vi "Control - Intake Air Measured.vi"(0 "MEP Desired [bar] (MAF w/ EGR Only)":sgl, 5 "Fuel [mg/cyc] (Fdbk)":sgl, 7 "Fuel Trim Integral Effort [mg/cyc] (VE Learn) (Fdbk) (optional)":sgl, 9 "Pre-Calculated EGR Mass Flow [kg/hr] (MAP Only)":sgl, 11 "Control Inputs":T1={"Engine Speed [RPM]"=0.0, "Engine Status"=enum."STALLED", "Load Control \nMode"=enum."High-Idle Governor", "dt(s)"=0.0, "Number of Cylinders"=0, "Engine Displacement [cc]"=0.0, "StoichAFR"=0.0, "Q.LHV Fuel [kJ/kg]"=0.0, "BattV PSU [V]"=0.0, "12V PSU [V]"=0.0, "5V PSU [V]"=0.0, "Pedal Position [%]"=0.0, "Oil Pressure [kPa]"=0.0, "Oil Temp [C]"=0.0, "Oil Level [%]"=0.0, "Engine Coolant Temp (ECT) [C]"=0.0, "Engine Coolant Pressure [kPa]"=0.0, "Rail Pressure [bar]"=0.0, "Fuel Pressure [kPa]"=0.0, "Fuel Temp [C]"=0.0, "Vacuum Pressure [kPa]"=0.0, "Throttle Position [%]"=0.0, "Cam1 Advance [CAD]"=0.0, "Cam2 Advance [CAD]"=0.0, "Cam3 Advance [CAD]"=0.0, "Cam4 Advance [CAD]"=0.0, "CA50 Control Output [CAD]"=[], "CA50 Control Output Valid"=[], "Intake Air Temp (IAT) [C]"=0.0, "Barometric Air Pressure [kPa]"=0.0, "Intake Air Rel. Humidity [%]"=0.0, "Mass Air Flow (MAF) [kg/hr]"=0.0, "Turbo Inlet Air Pressure [kPa]"=0.0, "Turbo Inlet Air Temp [C]"=0.0, "Turbo Outlet Air Pressure [kPa]"=0.0, "Turbo Outlet Air Temp [C]"=0.0, "CAC Outlet Pressure [kPa]"=0.0, "CAC Outlet Temp [C]"=0.0, "Intake Manifold Pressure (MAP) [kPa]"=0.0, "Intake Manifold Temp (MAT) [C]"=0.0, "Exhaust Manifold Pressure [kPa]"=0.0, "Exhaust Manifold Temp [C]"=0.0, "HighP EGR Cooler Outlet Pressure [kPa]"=0.0, "HighP EGR Cooler Outlet Temp [C]"=0.0, "HighP EGR Differential Pressure [kPa]"=0.0, "HighP EGR Valve Position [%]"=0.0, "Turbo Outlet Exhaust Pressure [kPa]"=0.0, "Turbo Outlet Exhaust Temp [C]"=0.0, "VGT Position 1 [%]"=0.0, "VGT Position 2 [%]"=0.0, "Turbo Speed 1 [RPM]"=0.0, "Turbo Speed 2 [RPM]"=0.0, "LowP EGR Differential Pressure [kPa]"=0.0, "LowP EGR Valve Position [%]"=0.0, "UEGO1Lambda"=0.0, "UEGO1_Hot"=FALSE, "UEGO2Lambda"=0.0, "UEGO2_Hot"=FALSE, "Knock Intensity"=[], "Knock"=[]} {"Knock Intensity" format="%.2f"; "CA50 Control Output [CAD]" format="%.2f"; "Exhaust Manifold Temp [C]" format="%#_6f"; "UEGO2Lambda" format="%.2f"; "Intake Manifold Temp (MAT) [C]" format="%#_6f"; "UEGO1Lambda" format="%.2f"}) -> (4 "Volumetric Efficiency [%]":sgl, 6 "Available Air Mass [mg/cyc]":sgl, 8 "Fresh Air Mass [mg/cyc]":sgl, 10 "Intake Charge Mass [mg/cyc]":sgl, 15 "EGR Mass [mg/cyc]":sgl)   [LabVIEW 2015, in "ECS-RT.lvlib"]
uses:
  ECS-RT.lvlib
  Typedefs/Control Inputs/Control Inputs.ctl
  Typedefs/EPT/Engine Status.ctl
  Typedefs/MISC/Load Control Mode.ctl
  Typedefs/MISC/Intake Charge Mode.ctl
  ECS-Shared.lvlib
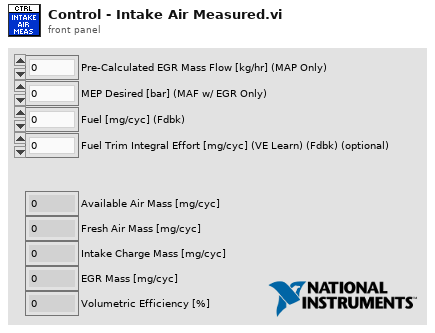
[diagram p1: front panel]
types:
  T1 = typedef "ECS-Shared.lvlib/Control Inputs.ctl" = cluster{"Engine Speed [RPM]":sgl, "Engine Status":T2, "Load Control \nMode":T3, "dt(s)":sgl, "Number of Cylinders":u8, "Engine Displacement [cc]":sgl, "StoichAFR":sgl, "Q.LHV Fuel [kJ/kg]":sgl, "BattV PSU [V]":sgl, "12V PSU [V]":sgl, "5V PSU [V]":sgl, "Pedal Position [%]":sgl, "Oil Pressure [kPa]":sgl, "Oil Temp [C]":sgl, "Oil Level [%]":sgl, "Engine Coolant Temp (ECT) [C]":sgl, "Engine Coolant Pressure [kPa]":sgl, "Rail Pressure [bar]":sgl, "Fuel Pressure [kPa]":sgl, "Fuel Temp [C]":sgl, "Vacuum Pressure [kPa]":sgl, "Throttle Position [%]":sgl, "Cam1 Advance [CAD]":sgl, "Cam2 Advance [CAD]":sgl, "Cam3 Advance [CAD]":sgl, "Cam4 Advance [CAD]":sgl, "CA50 Control Output [CAD]":sgl[], "CA50 Control Output Valid":bool[], "Intake Air Temp (IAT) [C]":sgl, "Barometric Air Pressure [kPa]":sgl, "Intake Air Rel. Humidity [%]":sgl, "Mass Air Flow (MAF) [kg/hr]":sgl, "Turbo Inlet Air Pressure [kPa]":sgl, "Turbo Inlet Air Temp [C]":sgl, "Turbo Outlet Air Pressure [kPa]":sgl, "Turbo Outlet Air Temp [C]":sgl, "CAC Outlet Pressure [kPa]":sgl, "CAC Outlet Temp [C]":sgl, "Intake Manifold Pressure (MAP) [kPa]":sgl, "Intake Manifold Temp (MAT) [C]":sgl, "Exhaust Manifold Pressure [kPa]":sgl, "Exhaust Manifold Temp [C]":sgl, "HighP EGR Cooler Outlet Pressure [kPa]":sgl, "HighP EGR Cooler Outlet Temp [C]":sgl, "HighP EGR Differential Pressure [kPa]":sgl, "HighP EGR Valve Position [%]":sgl, "Turbo Outlet Exhaust Pressure [kPa]":sgl, "Turbo Outlet Exhaust Temp [C]":sgl, "VGT Position 1 [%]":sgl, "VGT Position 2 [%]":sgl, "Turbo Speed 1 [RPM]":sgl, "Turbo Speed 2 [RPM]":sgl, "LowP EGR Differential Pressure [kPa]":sgl, "LowP EGR Valve Position [%]":sgl, "UEGO1Lambda":sgl, "UEGO1_Hot":bool, "UEGO2Lambda":sgl, "UEGO2_Hot":bool, "Knock Intensity":sgl[], "Knock":bool[]}
  T2 = typedef "ECS-Shared.lvlib/Engine Status.ctl" = enum16{"OFF", "STALLED", "CRANKING", "RUNNING", "ACCEL", "DECEL", "SAFE"}
  T3 = typedef "ECS-Shared.lvlib/Load Control Mode.ctl" = enum16{"No Governor", "Low-Idle Governor", "High-Idle Governor"}
  T4 = typedef "ECS-Shared.lvlib/Intake Charge Mode.ctl" = enum32{"MAF Only (No EGR)", "MAF Only (EGR)", "MAP Only (No EGR)", "MAP Only (EGR)", "MAF + MAP (EGR)"}
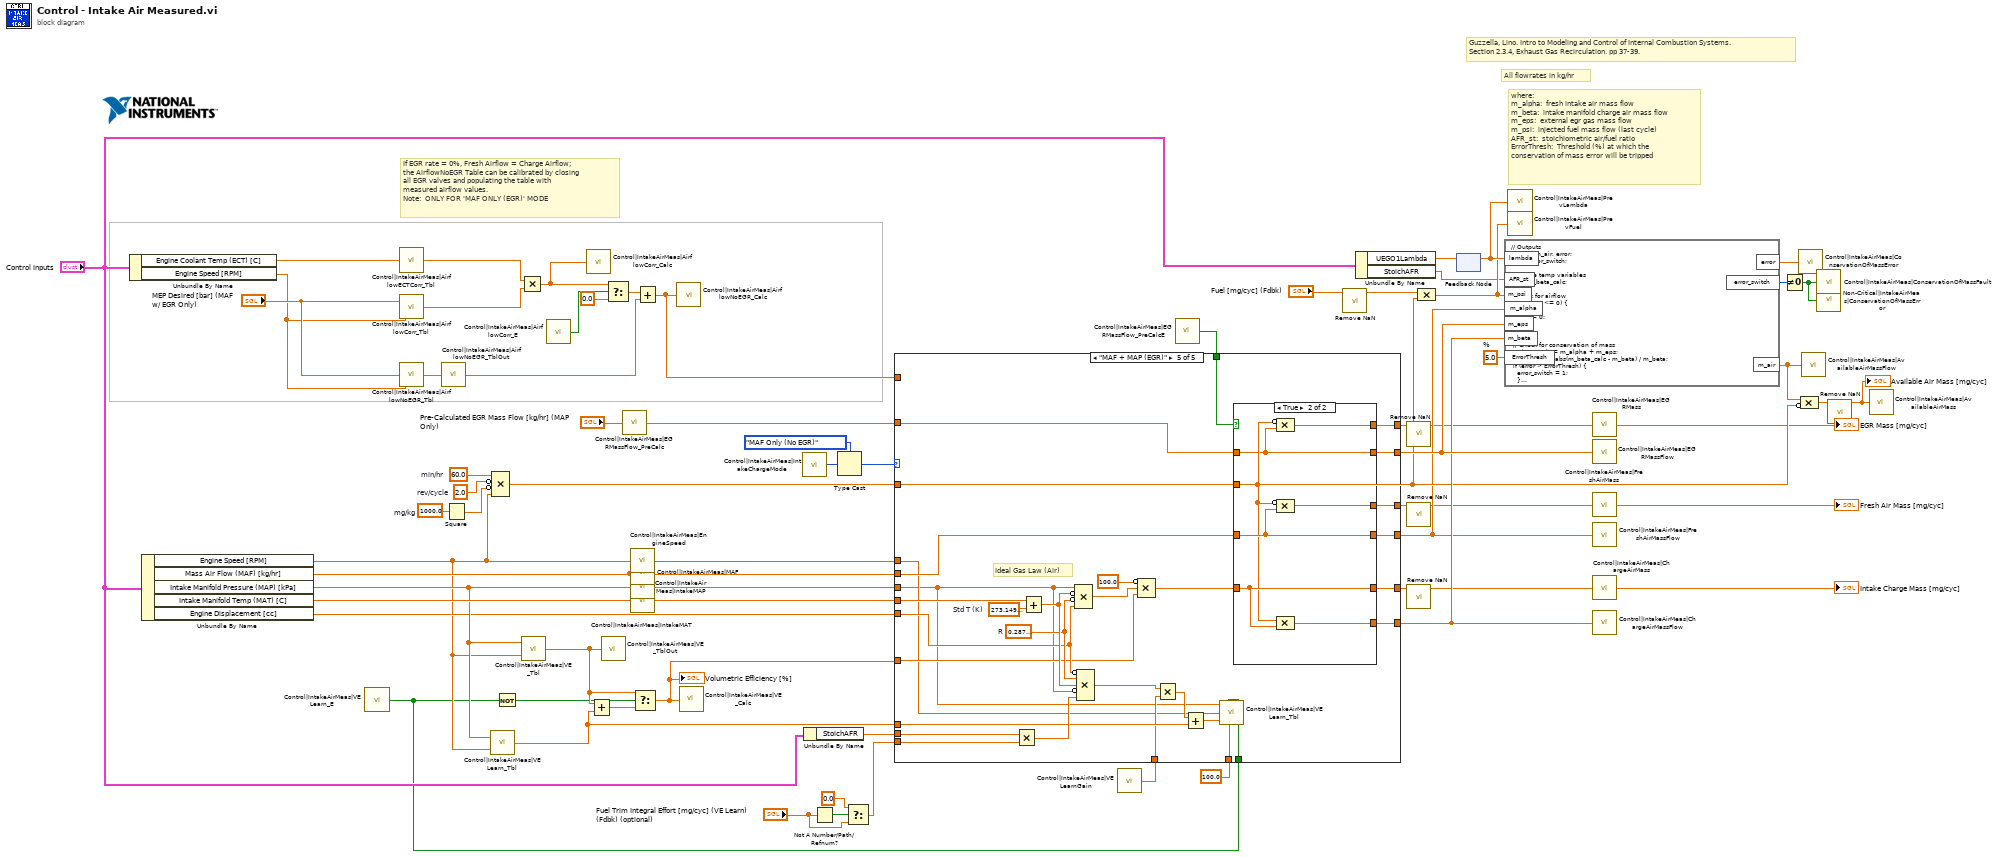
[diagram p0: block diagram]
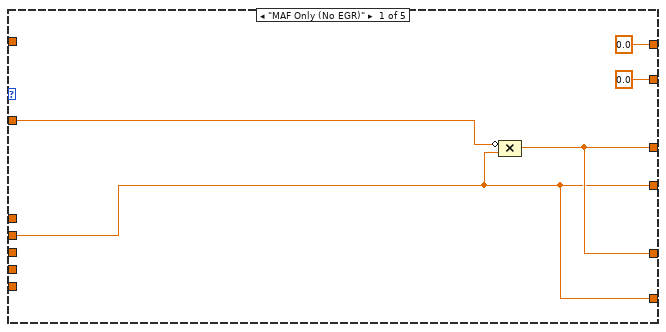
[diagram p2: hidden frame]
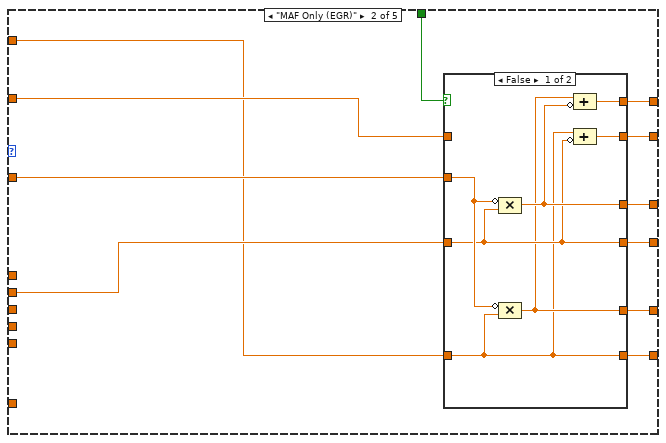
[diagram p3: hidden frame]
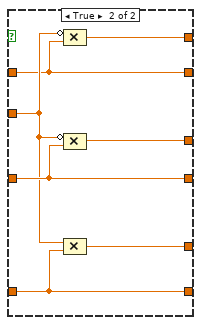
[diagram p4: hidden frame]
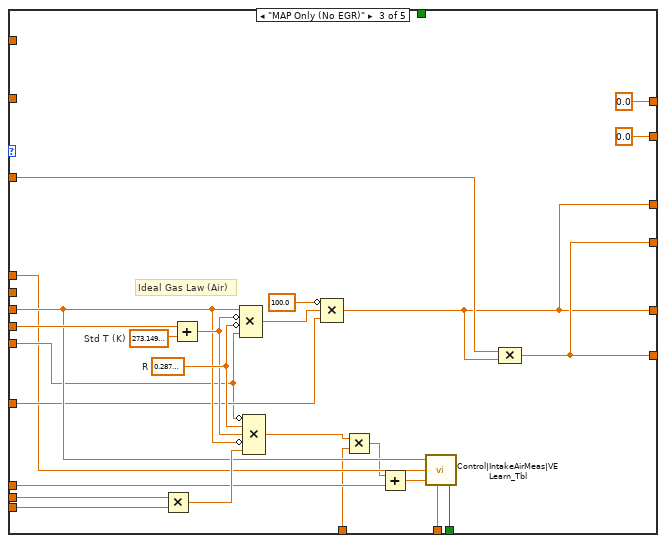
[diagram p5: hidden frame]
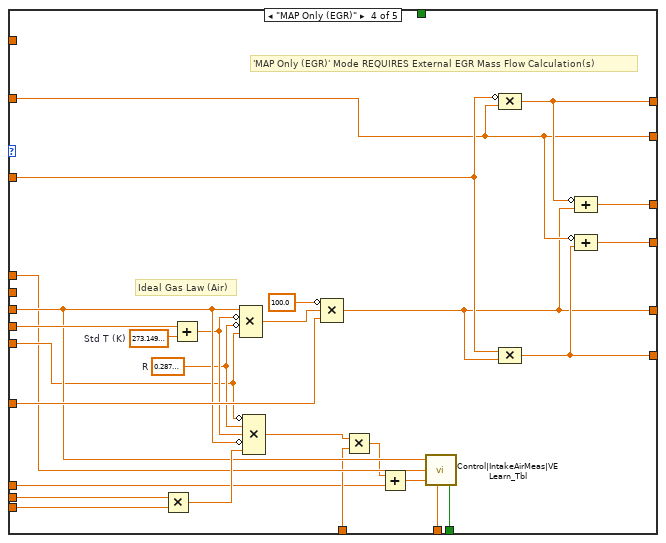
[diagram p6: hidden frame]
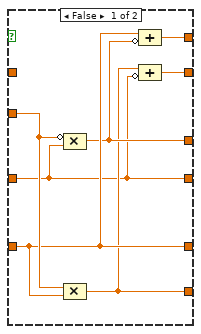
[diagram p7: hidden frame]
diagram:
  w40 = 5.0  # %
  w47 = sgl 60.0  # min/hr
  w48 = sgl 2.0  # rev/cycle
  w46 = sgl 1000.0  # mg/kg
  # "where:\nm_alpha:  fresh intake air mass flow\nm_beta:  intake manifold charge air mass flow\nm_eps:  external egr gas mass flow\nm_psi:  injected fuel mass flow (last cycle)\nAFR_st:  stoichiometric air/fuel ratio\nErrorThresh:  Threshold (%) at which the\nconservation of mass error will be tripped"
  # "All flowrates in kg/hr"
  # "Guzzella, Lino. Intro to Modeling and Control of Internal Combustion Systems.  \nSection 2.3.4, Exhaust Gas Recirculation. pp 37-39."
  # "If EGR rate = 0%, Fresh Airflow = Charge Airflow;\nthe AirflowNoEGR Table can be calibrated by closing\nall EGR valves and populating the table with\nmeasured airflow values.\nNote:  ONLY FOR 'MAF ONLY (EGR)' MODE"
  n1 = Unbundle By Name("Control Inputs") -> ("Engine Coolant Temp (ECT) [C]"=w52:sgl, "Engine Speed [RPM]"=w45:sgl)
  n2 = Unbundle By Name("Control Inputs") -> ("Engine Speed [RPM]"=w27:sgl, "Mass Air Flow (MAF) [kg/hr]"=w36:sgl, "Intake Manifold Pressure (MAP) [kPa]"=w29:sgl, "Intake Manifold Temp (MAT) [C]"=w35:sgl, "Engine Displacement [cc]"=w28:sgl)
  n3 = call "Control|IntakeAirMeas|VELearn_E"() -> ("Value"=w4:bool)
  n4 = call "Control|IntakeAirMeas|AirflowECTCorr_Tbl"("X Index"=w52) -> ("Y"=w57:sgl)
  n5 = call "Control|IntakeAirMeas|AirflowCorr_Tbl"("Y Index"=w45, "X Index"="MEP Desired [bar] (MAF w/ EGR Only)") -> ("Z"=w56:sgl)
  n6 = call "Control|IntakeAirMeas|AirflowNoEGR_Tbl"("Y Index"=w45, "X Index"="MEP Desired [bar] (MAF w/ EGR Only)") -> ("Z"=w59:sgl)
  n7 = call "Control|IntakeAirMeas|AirflowNoEGR_TblOut"("Value"=w59) -> ()
  n8 = Square(x=w46) -> (x^2=w49:sgl)
  n9 = call "Control|IntakeAirMeas|VELearn_Tbl"("Y Index"=w27, "X Index"=w29) -> ("Z"=w5:sgl)
  n10 = Compound Arithmetic op=MULTIPLY(w47, invert w48, invert w49, w27) -> (w26:sgl)
  n11 = Not(x=w4) -> (.not. x?=w3:bool)
  n12 = Multiply(x=w57, y=w56) -> (x*y=w58:sgl)
  n13 = call "Control|IntakeAirMeas|VE_Tbl"("Y Index"=w27, "X Index"=w29) -> ("Z"=w7:sgl)
  n14 = call "Control|IntakeAirMeas|AirflowCorr_E"() -> ("Value"=w54:bool)
  n15 = call "Control|IntakeAirMeas|AirflowCorr_Calc"("Value"=w58) -> ()
  n16 = Add(x=w7, y=w5) -> (x+y=w8:sgl)
  n17 = call "Control|IntakeAirMeas|VE_TblOut"("Value"=w7) -> ()
  n18 = Select(t=w58, s=w54, f=sgl 0.0) -> (s? t:f=w55:sgl)
  n19 = call "Control|IntakeAirMeas|EGRMassFlow_PreCalc"("Value"="Pre-Calculated EGR Mass Flow [kg/hr] (MAP Only)") -> ()
  n20 = call "Control|IntakeAirMeas|EngineSpeed"("Value"=w27) -> ()
  n21 = call "Control|IntakeAirMeas|MAF"("Value"=w36) -> ()
  n22 = call "Control|IntakeAirMeas|IntakeMAP"("Value"=w29) -> ()
  n23 = call "Control|IntakeAirMeas|IntakeMAT"("Value"=w35) -> ()
  n24 = Select(t=w7, s=w3, f=w8) -> (s? t:f=w21:sgl)
  "Volumetric Efficiency [%]" <- w21
  n25 = Add(x=w55, y=w59) -> (x+y=w51:sgl)
  n26 = call "Control|IntakeAirMeas|AirflowNoEGR_Calc"("Value"=w51) -> ()
  n27 = call "Control|IntakeAirMeas|VE_Calc"("Value"=w21) -> ()
  n28 = call "Control|IntakeAirMeas|IntakeChargeMode"() -> ("Value"=w62:u32)
  n29 = Unbundle By Name("Control Inputs") -> ("StoichAFR"=w10:sgl)
  n30 = Not A Number/Path/Refnum?(number/path/refnum="Fuel Trim Integral Effort [mg/cyc] (VE Learn) (Fdbk) (optional)") -> (NaN/Path/Refnum?=w19:bool)
  n31 = Type Cast(type=Intake_Charge_Mode."MAF Only (No EGR)" ("EGR Estimation Mode"), x=w62) -> (*(type *) &x=w60:T4)
  n32 = Select(t=sgl 0.0, s=w19, f="Fuel Trim Integral Effort [mg/cyc] (VE Learn) (Fdbk) (optional)") -> (s? t:f=w17:sgl)
  n33 = call "Control|IntakeAirMeas|VELearnGain"() -> ("Value"=w2:sgl)
  n34 = call "Control|IntakeAirMeas|EGRMassFlow_PreCalcE"() -> ("Value"=w33:bool)
  n35 = case shown="\"MAF + MAP (EGR)\"" w60 {
    tunnel: [sgl 0.0 ("EGR Mass Flow [kg/hr] (optional for MAF, MAF+MAP modes)") w74 sgl 0.0 ("EGR Mass Flow [kg/hr] (optional for MAF, MAF+MAP modes)") w135 w171] -> w42
    tunnel: [w63 w78 w111 w138 w175] -> w25
    tunnel: [w64 w76 w110 w139 w173] -> w24
    tunnel: w51 -> [_ w69 _ _ _]
    tunnel: [w63 w75 w111 w136 w172] -> w30
    tunnel: [w64 w77 w110 w134 w174] -> w22
    tunnel: [sgl 0.0 w73 sgl 0.0 w137 w170] -> w23
    tunnel: "Pre-Calculated EGR Mass Flow [kg/hr] (MAP Only)" -> [_ w72 _ w135 w169]
    tunnel: w26 -> [w67 w70 w114 w140 w168]
    tunnel: w36 -> [w63 w71 _ _ w147]
    tunnel: w29 -> [_ _ w102 w128 w145]
    tunnel: w35 -> [_ _ w109 w141 w159]
    tunnel: w28 -> [_ _ w100 w125 w160]
    tunnel: w21 -> [_ _ w101 w129 w158]
    tunnel: w33 -> [_ w68 _ _ w167]
    tunnel: w27 -> [_ _ w99 w124 w146]
    tunnel: w4 -> [_ _ w107 w131 w150]
    tunnel: sgl 100.0 ("Value") -> [_ _ w108 w130 w151]
    tunnel: w17 -> [_ _ w106 w132 w157]
    tunnel: w10 -> [_ _ w98 w123 w155]
    tunnel: w2 -> [_ _ w94 w121 w149]
    tunnel: w5 -> [_ _ w96 w118 w152]
    frame "MAF Only (No EGR)" {
      n36 = Compound Arithmetic op=MULTIPLY(invert w67, w63) -> (w64:sgl)
    }
    frame "MAF Only (EGR)" {
      n37 = case shown="False" w68 {
        tunnel: w71 -> [w81 w91]
        tunnel: w72 -> [_ w88]
        tunnel: [w81 w91] -> w78
        tunnel: [w80 w87] -> w77
        tunnel: w70 -> [w85 w89]
        tunnel: [w82 w92] -> w76
        tunnel: [w79 w86] -> w75
        tunnel: [w84 w88] -> w74
        tunnel: [w83 w90] -> w73
        tunnel: w69 -> [w79 w86]
        frame False {
          n38 = Compound Arithmetic op=MULTIPLY(invert w85, w81) -> (w82:sgl)
          n39 = Compound Arithmetic op=MULTIPLY(invert w85, w79) -> (w80:sgl)
          n40 = Compound Arithmetic op=ADD(w80, invert w82) -> (w83:sgl)
          n41 = Compound Arithmetic op=ADD(w79, invert w81) -> (w84:sgl)
        }
        frame True {
          n42 = Compound Arithmetic op=MULTIPLY(invert w89, w88) -> (w90:sgl)
          n43 = Compound Arithmetic op=MULTIPLY(invert w89, w91) -> (w92:sgl)
          n44 = Compound Arithmetic op=MULTIPLY(w89, w86) -> (w87:sgl)
        }
      }
    }
    frame "MAP Only (No EGR)" {
      w105 = sgl 0.287  # R
      w117 = sgl 273.15  # Std T (K)
      # "Ideal Gas Law (Air)"
      n45 = Multiply(x=w98, y=w106) -> (x*y=w103:sgl)
      n46 = Add(x=w109, y=w117) -> (x+y=w104:sgl)
      n47 = Compound Arithmetic op=MULTIPLY(w102, invert w104, invert w105, w100) -> (w115:sgl)
      n48 = Compound Arithmetic op=MULTIPLY(invert w100, w105, w104, invert w102, w103) -> (w95:sgl)
      n49 = Compound Arithmetic op=MULTIPLY(invert sgl 100.0 ("y"), w115, w101) -> (w110:sgl)
      n50 = Multiply(x=w95, y=w94) -> (x*y=w93:sgl)
      n51 = Add(x=w93, y=w96) -> (x+y=w97:sgl)
      n52 = call "Control|IntakeAirMeas|VELearn_Tbl"("X"=w102, "Adapt"=w107, "Y"=w99, "Z"=w97, "%/100"=w108) -> ()  [unwired: 1 in]
      n53 = Compound Arithmetic op=MULTIPLY(w114, w110) -> (w111:sgl)
    }
    frame "MAP Only (EGR)" {
      w126 = sgl 0.287  # R
      w144 = sgl 273.15  # Std T (K)
      # "'MAP Only (EGR)' Mode REQUIRES External EGR Mass Flow Calculation(s)"
      # "Ideal Gas Law (Air)"
      n54 = Multiply(x=w123, y=w132) -> (x*y=w133:sgl)
      n55 = Add(x=w141, y=w144) -> (x+y=w127:sgl)
      n56 = Compound Arithmetic op=MULTIPLY(w128, invert w127, invert w126, w125) -> (w142:sgl)
      n57 = Compound Arithmetic op=MULTIPLY(invert w125, w126, w127, invert w128, w133) -> (w120:sgl)
      n58 = Compound Arithmetic op=MULTIPLY(invert sgl 100.0 ("y"), w142, w129) -> (w134:sgl)
      n59 = Multiply(x=w120, y=w121) -> (x*y=w119:sgl)
      n60 = Add(x=w119, y=w118) -> (x+y=w122:sgl)
      n61 = call "Control|IntakeAirMeas|VELearn_Tbl"("X"=w128, "Adapt"=w131, "Y"=w124, "Z"=w122, "%/100"=w130) -> ()  [unwired: 1 in]
      n62 = Compound Arithmetic op=MULTIPLY(invert w140, w135) -> (w137:sgl)
      n63 = Compound Arithmetic op=MULTIPLY(w140, w134) -> (w136:sgl)
      n64 = Compound Arithmetic op=ADD(invert w137, w134) -> (w139:sgl)
      n65 = Compound Arithmetic op=ADD(invert w135, w136) -> (w138:sgl)
    }
    frame "MAF + MAP (EGR)" {
      w161 = sgl 0.287  # R
      w166 = sgl 273.15  # Std T (K)
      # "Ideal Gas Law (Air)"
      # "Ideal Gas Law (Air)"
      n66 = Multiply(x=w155, y=w157) -> (x*y=w163:sgl)
      n67 = Add(x=w159, y=w166) -> (x+y=w162:sgl)
      n68 = Compound Arithmetic op=MULTIPLY(w145, invert w162, invert w161, w160) -> (w164:sgl)
      n69 = Compound Arithmetic op=MULTIPLY(invert w160, w161, w162, invert w145, w163) -> (w148:sgl)
      n70 = Compound Arithmetic op=MULTIPLY(invert sgl 100.0 ("y"), w164, w158) -> (w156:sgl)
      n71 = Multiply(x=w148, y=w149) -> (x*y=w153:sgl)
      n72 = Add(x=w153, y=w152) -> (x+y=w154:sgl)
      n73 = call "Control|IntakeAirMeas|VELearn_Tbl"("X"=w145, "Adapt"=w150, "Y"=w146, "Z"=w154, "%/100"=w151) -> ()  [unwired: 1 in]
      n74 = case shown="True" w167 {
        tunnel: w156 -> [w179 w187]
        tunnel: w147 -> [w176 w186]
        tunnel: w169 -> [_ w183]
        tunnel: [w176 w186] -> w175
        tunnel: [w179 w187] -> w174
        tunnel: w168 -> [w182 w184]
        tunnel: [w178 w189] -> w173
        tunnel: [w177 w188] -> w172
        tunnel: [w181 w183] -> w171
        tunnel: [w180 w185] -> w170
        frame False {
          n75 = Compound Arithmetic op=MULTIPLY(invert w182, w176) -> (w178:sgl)
          n76 = Compound Arithmetic op=MULTIPLY(w182, w179) -> (w177:sgl)
          n77 = Compound Arithmetic op=ADD(w179, invert w178) -> (w180:sgl)
          n78 = Compound Arithmetic op=ADD(w177, invert w176) -> (w181:sgl)
        }
        frame True {
          n79 = Compound Arithmetic op=MULTIPLY(invert w184, w183) -> (w185:sgl)
          n80 = Compound Arithmetic op=MULTIPLY(invert w184, w186) -> (w189:sgl)
          n81 = Compound Arithmetic op=MULTIPLY(w184, w187) -> (w188:sgl)
        }
      }
    }
  }
  n82 = call "Remove NaN.vi"("Value In"="Fuel [mg/cyc] (Fdbk)") -> ("Value Out"=w15:sgl)  [unwired: 10 in]
  n83 = Unbundle By Name("Control Inputs") -> ("UEGO1Lambda"=w41:sgl, "StoichAFR"=w1:sgl)
  n84 = call "Remove NaN.vi"("Value In"=w23) -> ("Value Out"=w14:sgl)  [unwired: 10 in]
  "EGR Mass [mg/cyc]" <- w14
  n85 = call "Remove NaN.vi"("Value In"=w24) -> ("Value Out"=w13:sgl)  [unwired: 10 in]
  "Fresh Air Mass [mg/cyc]" <- w13
  n86 = call "Remove NaN.vi"("Value In"=w22) -> ("Value Out"=w12:sgl)  [unwired: 10 in]
  "Intake Charge Mass [mg/cyc]" <- w12
  n87 = Compound Arithmetic op=MULTIPLY(w15, w26) -> (w31:sgl)
  n88 = feedback-in #1(w41) -> ()
  n89 = feedback #1() -> (w32:sgl)  [unwired: 1 in]
  n90 = formula code="// Outputs\nfloat32 m_air, error;\nuInt8 error_switch;\n\n// Create temp variables\nfloat m_beta_calc;\n\n//Check for airflow\nif (m_beta <= 0) {\n error = 0;\n m_air = 0;\n }\nelse {\n\n // Check for conservation of mass\n m_beta_calc = m_alpha + m_eps;\n error = 100 * abs(m_beta_calc - m_beta) / m_beta;\n if (error > ErrorThresh) {\n   error_switch = 1;\n   }\n else {\n   error_switch = 0;\n   }\n\n // Calculate Available air mass flow\n if (lambda < 1) {\n   m_air = m_alpha;\n    }\n else {\n   m_air = m_alpha + ((m_eps*(lambda-1)*AFR_st*m_psi)/(m_beta+m_psi));\n   }\n }"("m_psi"=w31, "m_beta"=w30, "lambda"=w32, "AFR_st"=w1, "m_eps"=w42, "m_alpha"=w25, "ErrorThresh"=w40) -> ("m_air"=w44:sgl, "error_switch"=w38:u8, "error"=w39:sgl)
  n91 = call "Control|IntakeAirMeas|PrevLambda"("Value"=w32) -> ()
  n92 = call "Control|IntakeAirMeas|PrevFuel"("Value"=w31) -> ()
  n93 = call "Control|IntakeAirMeas|EGRMass"("Value"=w14) -> ()
  n94 = call "Control|IntakeAirMeas|EGRMassFlow"("Value"=w42) -> ()
  n95 = call "Control|IntakeAirMeas|FreshAirMass"("Value"=w13) -> ()
  n96 = call "Control|IntakeAirMeas|FreshAirMassFlow"("Value"=w25) -> ()
  n97 = call "Control|IntakeAirMeas|ChargeAirMass"("Value"=w12) -> ()
  n98 = call "Control|IntakeAirMeas|ChargeAirMassFlow"("Value"=w30) -> ()
  n99 = Not Equal To 0?(x=w38) -> (x != 0?=w37:bool)
  n100 = call "Control|IntakeAirMeas|ConservationOfMassError"("Value"=w39) -> ()
  n101 = Compound Arithmetic op=MULTIPLY(w44, invert w26) -> (w43:sgl)
  n102 = call "Control|IntakeAirMeas|AvailableAirMassFlow"("Value"=w44) -> ()
  n103 = call "Control|IntakeAirMeas|ConservationOfMassFault"("Value"=w37) -> ()
  n104 = call "Non-Critical|IntakeAirMeas|ConservationOfMassError"("Fault"=w37) -> ()  [unwired: 2 in]
  n105 = call "Remove NaN.vi"("Value In"=w43) -> ("Value Out"=w11:sgl)  [unwired: 10 in]
  "Available Air Mass [mg/cyc]" <- w11
  n106 = call "Control|IntakeAirMeas|AvailableAirMass"("Value"=w11) -> ()
